vi "WS1040_PIC_Initialize.vi"(0 "COM_In":refnum<visa-resource-name>, 1 "baud rate (9600)":u32=9600, 2 "stop bits (10: 1 bit)":u16(ring)=10 items=["1.0"=10, "1.5"=15, "2.0"=20], 3 "parity (0:none)":enum16{"None", "Odd", "Even", "Mark", "Space"}(ring), 4 "flow control (0:none)":u16(ring) items=["None", "XON/XOFF", "RTS/CTS", "XON/XOFF & RTS/CTS", "DTR/DSR", "XON/XOFF & DTR/DSR"], 5 "error in (no error)":errorcluster, 6 "timeout (10sec)":u32=10000, 7 "data bits (8)":u16=8 min=5 max=8 step=1) -> (14 "COM_Out":refnum<visa-resource-name>, 19 "error out":errorcluster)   [LabVIEW 2017]
uses:
  <vilib>/Instr/_visa.llb/VISA Configure Serial Port (Instr).vi
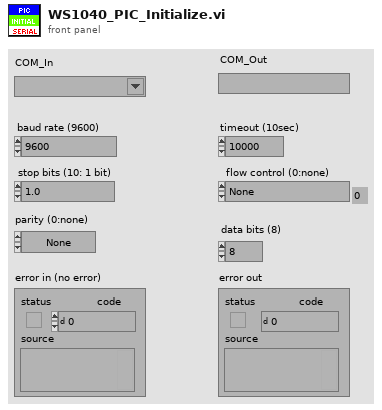
[diagram p1: front panel]
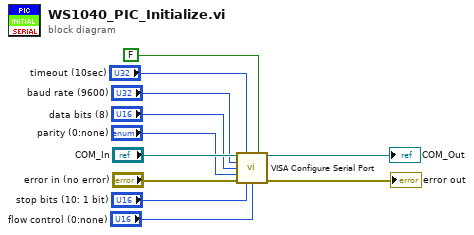
[diagram p0: block diagram]
diagram:
  n1 = call-poly "VISA Configure Serial Port"("VISA resource name"="COM_In", "timeout (10sec)"="timeout (10sec)", "Enable Termination\nChar (T)"=FALSE ("Enable Termination\nChar (T)"), "baud rate (9600)"="baud rate (9600)", "data bits (8)"="data bits (8)", "parity (0:none)"="parity (0:none)", "error in (no error)"="error in (no error)", "stop bits (10: 1 bit)"="stop bits (10: 1 bit)", "flow control (0:none)"="flow control (0:none)") -> ("VISA resource name out"=→"COM_Out":refnum<visa-resource-name>, "error out"=→"error out":errorcluster)  [unwired: 5 in]
